vi "Set and Print Serial Wire Mode to Console.vi"(8 "error in (no error)":errorcluster, 10 "Wire Mode":i16, 11 "VISA Refnum in":refnum<visa-resource-name>) -> (0 "error out":errorcluster, 3 "VISA Refnum out":refnum<visa-resource-name>)   [LabVIEW 2021, in "Modbus Master Engine.lvlib"]
uses:
  Modbus Master Engine.lvlib
  <vilib>/NI VeriStand/Custom Device Tools/Custom Device Utility Library/Custom Device Utility Library.lvlib
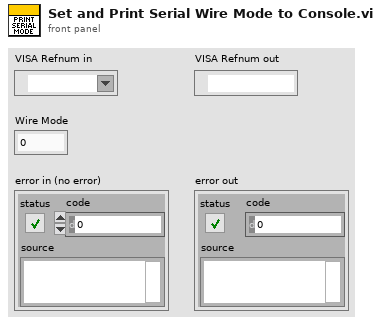
[diagram p1: front panel]
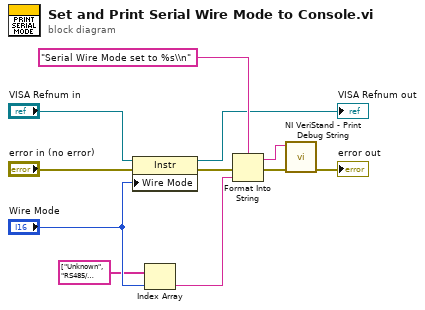
[diagram p0: block diagram]
diagram:
  n1 = property class="Instr"(reference="VISA Refnum in", error in="error in (no error)", "Wire Mode"="Wire Mode") -> (reference out=→"VISA Refnum out":refnum<visa-resource-name>, error out=w7:errorcluster)
  n2 = Index Array(array=string[] ["Unknown", "RS485/Wire4", "RS485/Wire2-EchoDTR", "RS485/Wire2-CtrlDTR", "RS485/Wire2-Auto", "RS232/DTE", "RS232/DCE", "RS232/AUTO"] ("Strings []"), index="Wire Mode") -> (element=w11:string)
  n3 = Format Into String(format string="Serial Wire Mode set to %s\\n", error in=w7, w11) -> (resulting string=w5:string, error out=w8:errorcluster)  [unwired: 1 in]
  n4 = call <vilib>:"NI VeriStand - Print Debug String.vi"("error in (no error)"=w8, "Message"=w5) -> ("error out"=→"error out":errorcluster)  [unwired: 9 in]
